vi "Device Clear.vi"(8 "error in (no error)":errorcluster, 11 "VISA Resource Name":refnum<visa-resource-name>) -> (0 "error out":errorcluster, 3 "VISA Resource Out":refnum<visa-resource-name>)   [LabVIEW 2024, in "Lake Shore 336.lvlib"]
doc: "Device clear is an IEEE-488 low-level bus message. It clears Model 336 interface activity and puts it into a bus idle state."
uses:
  Lake Shore 336.lvlib
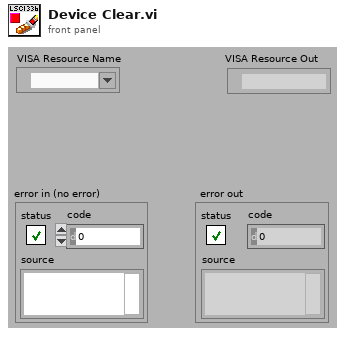
[diagram p1: front panel]
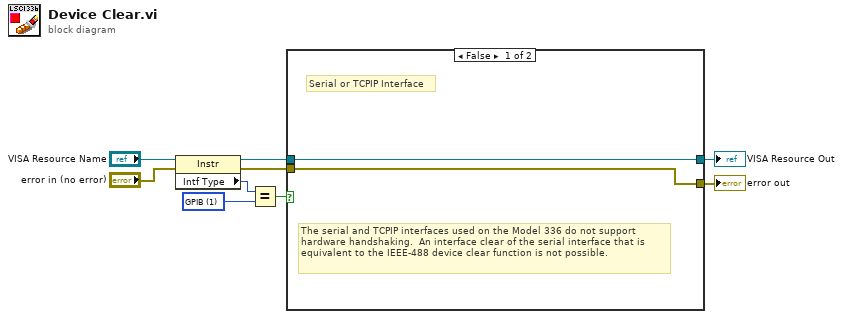
[diagram p0: block diagram]
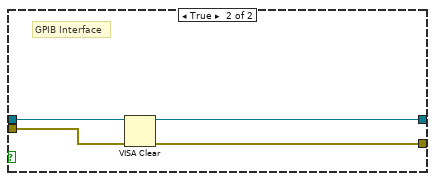
[diagram p2: hidden frame]
diagram:
  w7 = u16 1 items=["GPIB"=1, "VXI"=2, "GPIB-VXI"=3, "Serial"=4, "PXI"=5, "TCPIP"=6, "USB"=7] ("Interface Information:Interface Type")
  n1 = property class="Instr"(reference="VISA Resource Name", error in="error in (no error)") -> (reference out=w3:refnum<visa-resource-name>, error out=w2:errorcluster, "Intf Type"=w6:u16)
  n2 = Equal?(x=w6, y=w7) -> (x = y?=w1:bool)
  n3 = case shown="False" w1 {
    tunnel: w2 -> [w11 w12]
    tunnel: [w10 w14] -> w9
    tunnel: [w11 w13] -> w8
    tunnel: w3 -> [w10 w15]
    frame False {
      # "The serial and TCPIP interfaces used on the Model 336 do not support hardware handshaking.  An interface clear of the serial interface that is equivalent to the IEEE-488 device clear function is not possible."
      # "Serial or TCPIP Interface"
    }
    frame True {
      # "GPIB Interface"
      n4 = VISA Clear(VISA resource name=w15, error in (no error)=w12) -> (VISA resource name out=w14:refnum<visa-resource-name>, error out=w13:errorcluster)
    }
  }
  "VISA Resource Out" <- w9
  "error out" <- w8
